vi "GetDefaultParams.vi"(8 "error in (no error)":errorcluster, 10 "config file path":path, 11 "Class In":refnum<class "NISTFGenPluginsBase.lvclass">) -> (0 "error out":errorcluster, 3 "Class Out":refnum<class "NISTFGenPluginsBase.lvclass">)   [LabVIEW 2014, in "FGenPlugins.lvlib" / "NISTFGenPluginsBase.lvclass"]
uses:
  NISTFGenPluginsBase.lvclass
  TypeDef/ResourceNameParams.ctl
  TypeDef/ArbWfrmParams.ctl
  TypeDef/StdWaveformParams.ctl
  TypeDef/RefClkSourceParams.ctl
  TypeDef/ChannelParamElement.ctl
  <userlib>/NIST/BaseClasses/BasePlugin_class/BasePlugin.lvclass/BasePlugin.ctl
  <userlib>/NIST/BaseClasses/BasePlugin_class/Accessors/Write PluginIniFilePath.vi
  <vilib>/Utility/config.llb/NI_LVConfig.lvlib
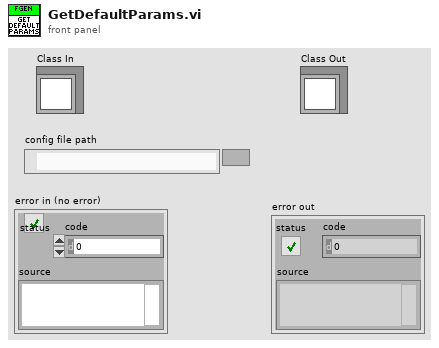
[diagram p1: front panel]
types:
  T1 = typedef "FGenPlugins.lvlib/NISTFGenPluginsBase.lvclass/RefClkSourceParams.ctl" = cluster{"eRefClk":u16}
  T2 = typedef "FGenPlugins.lvlib/NISTFGenPluginsBase.lvclass/StdWaveformParams.ctl" = cluster{"eWaveform":u16, "dAmplitude":dbl, "dDcOffset":dbl, "dFrequency":dbl, "dStartPhase":dbl, "dSampleRate":dbl, "dNumSamples":dbl}
  T3 = typedef "FGenPlugins.lvlib/NISTFGenPluginsBase.lvclass/ArbWfrmParams.ctl" = cluster{"sWfrmHandle":string, "iSize":i32, "dData":dbl[], "dGain":dbl, "dOffset":dbl, "dSampleRate":dbl}
  T4 = cluster{"eTrigger":u16, "eEdge":u16, "sSource":string}
  T5 = typedef "FGenPlugins.lvlib/NISTFGenPluginsBase.lvclass/ResourceNameParams.ctl" = cluster{"Handle":string}
  T6 = typedef "NI_LVConfig.lvlib/Config Data RefNum.ctl" = refnum<k1>
  T7 = typedef "FGenPlugins.lvlib/NISTFGenPluginsBase.lvclass/ChannelParamElement.ctl" = cluster{"sName":string, "eOperateMode":u16, "bEnabled":bool, "eOutputMode":u16, "iIndex":i32, "iNameBufferSize":i32, "fGain":dbl}
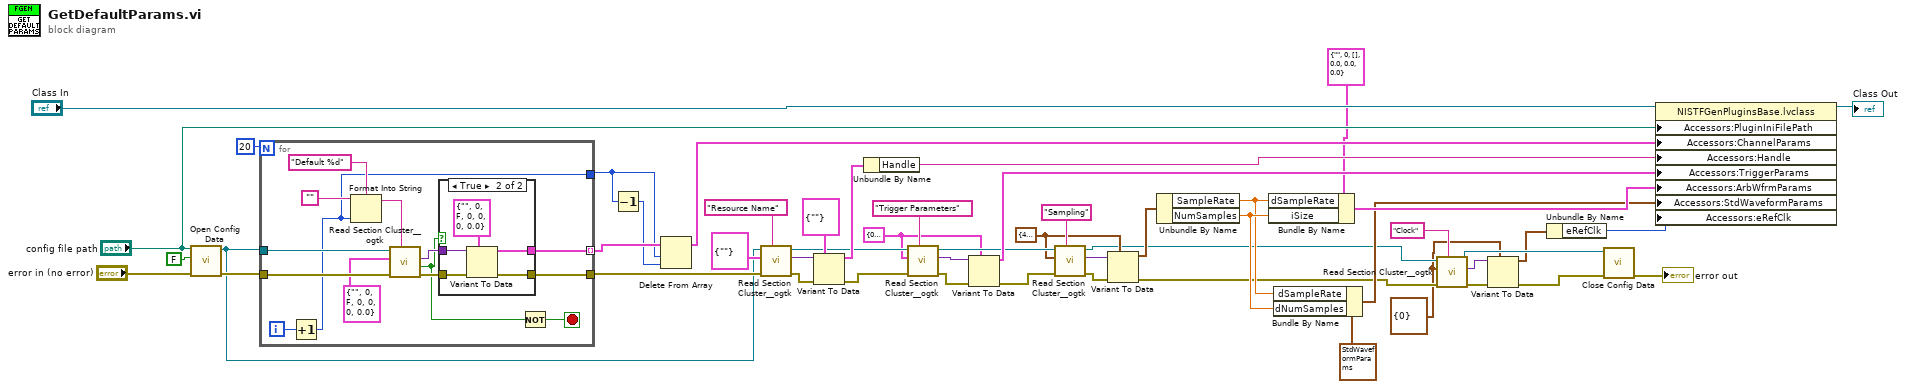
[diagram p0: block diagram]
diagram:
  w3 = T1 {"eRefClk"=0} ("RefClkSourceParams")
  w18 = cluster{"SampleRate":dbl, "NumSamples":dbl} {"SampleRate"=4800.0, "NumSamples"=4800.0}
  w21 = T4 {"eTrigger"=0, "eEdge"=10280, "sSource"=""} ("TriggerParams")
  n1 = call <vilib>:"Open Config Data.vi"("error in (no error)"="error in (no error)", "create file if necessary (T)"=FALSE, "configuration file path"="config file path") -> ("error out"=w50:errorcluster, "refnum"=w41:T6)  [unwired: 6 in, 1 out]
  n2 = for {
    N: 20 -> [_]
    tunnel: w41 -> [w65]
    tunnel: w50 -> [w64]
    tunnel: [w55] -> w39 mode=indexing
    tunnel: [w54] -> w42
    tunnel: [w52] -> w38
    i -> [w59]
    stop <- w58 stop-if-true
    n3 = Increment(x=w59) -> (x+1=w52:i32)
    n4 = Format Into String(format string="Default %d", initial string="", w52) -> (resulting string=w60:string)  [unwired: 1 in, 1 out]
    n5 = call <userlib>:"Read Section Cluster__ogtk.vi"("section (optional)"=w60, "error in (no error)"=w64, "Section Formatted Cluster Type"=T7 {"sName"="", "eOperateMode"=0, "bEnabled"=FALSE, "eOutputMode"=0, "iIndex"=0, "iNameBufferSize"=0, "fGain"=0.0} ("ChannelParamElement"), "refnum"=w65) -> ("error out"=w56:errorcluster, "all found?"=w53:bool, "Section Formatted Cluster"=w57:variant)  [unwired: 3 in, 2 out]
    n6 = case shown="True" w53 {
      tunnel: w57 -> [_ w70]
      tunnel: w56 -> [w66 w69]
      tunnel: [_ w68] -> w55
      tunnel: [w66 w67] -> w54
      frame False {
      }
      frame True {
        n7 = Variant To Data(error in=w69, type=T7 {"sName"="", "eOperateMode"=0, "bEnabled"=FALSE, "eOutputMode"=0, "iIndex"=0, "iNameBufferSize"=0, "fGain"=0.0} ("ChannelParamElement"), Variant=w70) -> (data=w68:T7, error out=w67:errorcluster)
      }
    }
    n8 = Not(x=w53) -> (.not. x?=w58:bool)
  }
  n9 = Decrement(x=w38) -> (x-1=w37:i32)
  n10 = Delete From Array(array=w39, length=w38, index=w37) -> (array with subset deleted=w27:T7[])  [unwired: 1 out]
  n11 = call <userlib>:"Read Section Cluster__ogtk.vi"("section (optional)"="Resource Name", "error in (no error)"=w42, "Section Formatted Cluster Type"=T5 {"Handle"=""} ("ResourceName"), "refnum"=w41) -> ("error out"=w47:errorcluster, "Section Formatted Cluster"=w46:variant, "dup refnum"=w35:T6)  [unwired: 3 in, 2 out]
  n12 = Variant To Data(error in=w47, type=T5 {"Handle"=""} ("ResourceName"), Variant=w46) -> (data=w43:T5, error out=w34:errorcluster)
  n13 = Unbundle By Name(w43) -> ("Handle"=w26:string)
  n14 = call <userlib>:"Read Section Cluster__ogtk.vi"("section (optional)"="Trigger Parameters", "error in (no error)"=w34, "Section Formatted Cluster Type"=w21, "refnum"=w35) -> ("error out"=w31:errorcluster, "Section Formatted Cluster"=w32:variant, "dup refnum"=w23:T6)  [unwired: 3 in, 2 out]
  n15 = Variant To Data(error in=w31, type=w21, Variant=w32) -> (data=w25:T4, error out=w24:errorcluster)
  n16 = call <userlib>:"Read Section Cluster__ogtk.vi"("section (optional)"="Sampling" ("section"), "error in (no error)"=w24, "Section Formatted Cluster Type"=w18, "refnum"=w23) -> ("error out"=w19:errorcluster, "Section Formatted Cluster"=w20:variant, "dup refnum"=w6:T6)  [unwired: 3 in, 2 out]
  n17 = Variant To Data(error in=w19, type=w18, Variant=w20) -> (data=w17:cluster{"SampleRate":dbl, "NumSamples":dbl}, error out=w8:errorcluster)
  n18 = Unbundle By Name(w17) -> ("SampleRate"=w12:dbl, "NumSamples"=w13:dbl)
  n19 = Bundle By Name(cluster=T3 {"sWfrmHandle"="", "iSize"=0, "dData"=[], "dGain"=0.0, "dOffset"=0.0, "dSampleRate"=0.0} ("ArbWfrmParams"), "dSampleRate"=w12, "iSize"=w13) -> (w14:T3)
  n20 = Bundle By Name(cluster=T2 {"eWaveform"=0, "dAmplitude"=0.1, "dDcOffset"=0.0, "dFrequency"=1000.0, "dStartPhase"=1000.0, "dSampleRate"=1000.0, "dNumSamples"=1000.0} ("StdWaveformParams"), "dSampleRate"=w12, "dNumSamples"=w13) -> (w11:T2)
  n21 = call <userlib>:"Read Section Cluster__ogtk.vi"("section (optional)"="Clock", "error in (no error)"=w8, "Section Formatted Cluster Type"=w3, "refnum"=w6) -> ("error out"=w10:errorcluster, "Section Formatted Cluster"=w9:variant, "dup refnum"=w5:T6)  [unwired: 3 in, 2 out]
  n22 = Variant To Data(error in=w10, type=w3, Variant=w9) -> (data=w1:T1, error out=w7:errorcluster)
  n23 = Unbundle By Name(w1) -> ("eRefClk"=w2:u16)
  n24 = call <vilib>:"Close Config Data.vi"("error in (no error)"=w7, "refnum"=w5) -> ("error out"=→"error out":errorcluster)  [unwired: 8 in, 1 out]
  n25 = property class="NISTFGenPluginsBase.lvclass"(reference="Class In", "Accessors:PluginIniFilePath"="config file path", "Accessors:ChannelParams"=w27, "Accessors:Handle"=w26, "Accessors:TriggerParams"=w25, "Accessors:ArbWfrmParams"=w14, "Accessors:StdWaveformParams"=w11, "Accessors:eRefClk"=w2) -> (reference out=→"Class Out":refnum<class "NISTFGenPluginsBase.lvclass">)  [unwired: 1 in, 1 out]
